vi "Timer data class VI - retrieve times.vi"(0 "Timer in":refnum<class "Timer.lvclass">, 11 "error in (no error)":errorcluster) -> (4 "Timer out":refnum<class "Timer.lvclass">, 6 "Milliseconds":u32, 8 "Time 1":u32, 10 "Time 2":u32, 15 "error out":errorcluster)   [LabVIEW 2010, in "Timer.lvclass"]
uses:
  Timer.lvclass
  Timer.lvclass/Timer.ctl
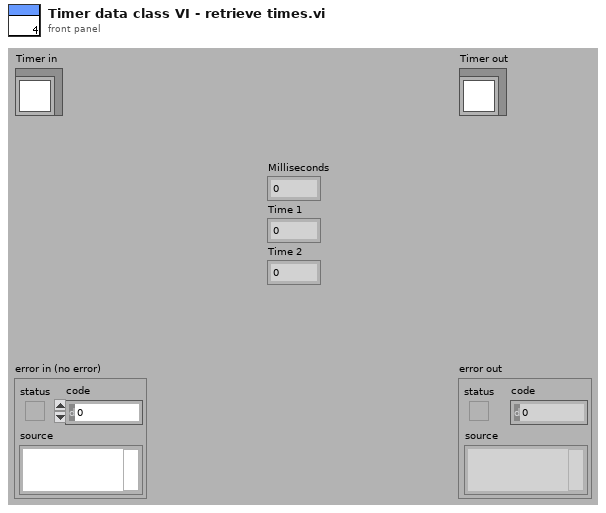
[diagram p1: front panel]
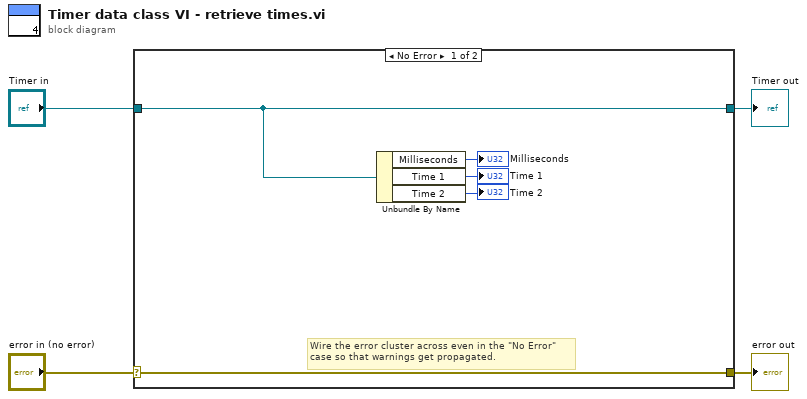
[diagram p0: block diagram]
diagram:
  n1 = case shown="No Error" "error in (no error)" {
    selector: "error in (no error)" -> [w9 w11]
    tunnel: [w9 w11] -> w3
    tunnel: [w8 w10] -> w1
    tunnel: "Timer in" -> [w8 w10]
    frame No Error {
      # "Wire the error cluster across even in the \"No Error\"\ncase so that warnings get propagated."
      n2 = Unbundle By Name(w8) -> ("Milliseconds"=→"Milliseconds":u32, "Time 1"=→"Time 1":u32, "Time 2"=→"Time 2":u32)
    }
    frame Error {
    }
  }
  "error out" <- w3
  "Timer out" <- w1
